vi "RT IO Module.vi"(0 "FPGA VI Reference In":refnum<k20>, 3 "Error In":errorcluster) -> (4 "Accelerometer":cluster{"Z":i16, "Y":i16, "X":i16}, 5 "Ultrasuond":cluster{"US BK":i16, "US FR":i16, "US FL":i16}, 6 "IR":cluster{"1":bool, "2":bool}, 7 "FPGA VI Reference Out":refnum<k20>, 8 "PIR":bool, 9 "Button":bool, 10 "Error Out":errorcluster)   [LabVIEW 2015]
uses:
  <vilib>/Utility/error.llb/Error Cluster From Error Code.vi
  <vilib>/rvi/errors/niLvFpgaAdjustHostInterfaceError.vi
  <vilib>/rvi/interface/nirviReadWriteControl/nirviReadWriteControl.xnode
  NiFpgaLv.dll
  <vilib>/rvi/interface/Simulation/niFpgaSimulationCallBeginRW.vi
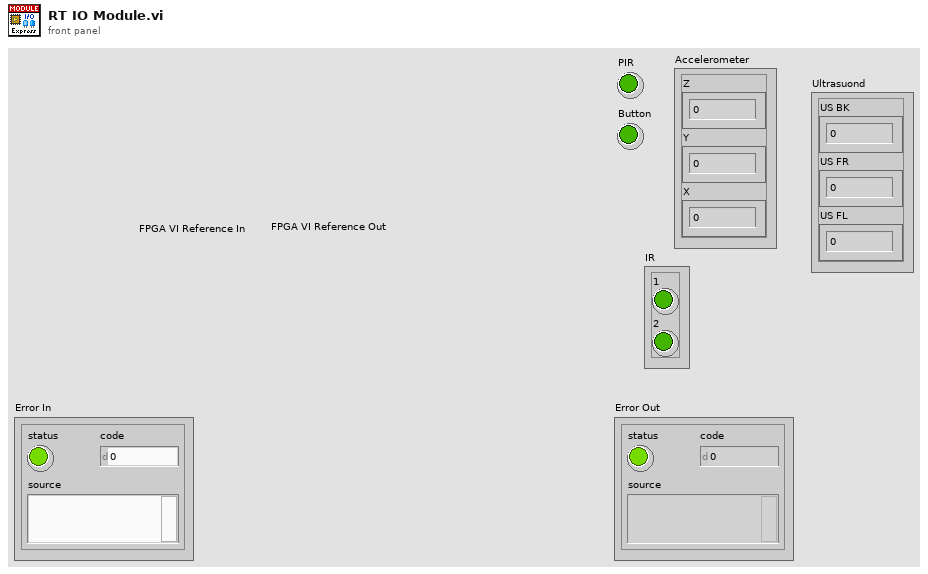
[diagram p1: front panel]
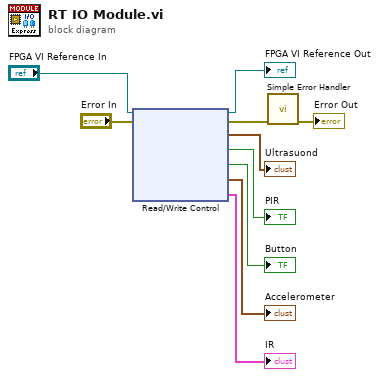
[diagram p0: block diagram]
diagram:
  n1 = xnode "Read/Write Control"("FPGA VI Reference In"="FPGA VI Reference In", "error in"="Error In") -> ("FPGA VI Reference Out"=→"FPGA VI Reference Out":refnum<k20>, "error out"=w5:errorcluster, "Ultrasuond"=→"Ultrasuond":cluster{"US BK":u32, "US FR":u32, "US FL":u32}, "PIR"=→"PIR":bool, "Button"=→"Button":bool, "Accelerometer"=→"Accelerometer":cluster{"Z":i16, "Y":i16, "X":i16}, "IR"=→"IR":cluster{"1":bool, "2":bool})
  n2 = call <vilib>:"Simple Error Handler.vi"("error in (no error)"=w5) -> ("error out"=→"Error Out":errorcluster)  [unwired: 4 in, 4 out]
